vi "rsscope_core_global.vi"() -> ()   [LabVIEW 2018] (continued)
"Supported Models"="", "Instrument Options"="", "Flags"=0, "Help"="Adds additional time limitation to the pattern definition.\n\nAvailable Repeated Capabilities:\nNone\n\nRemote-control command(s):\nTRIGger<m>:PATTern:MODE"}, {"Level"=3, "Class Only"=FALSE, "Identifier"="RSSCOPE_ATTR_PATTERN_TIMEOUT_MODE", "Descriptive Name"="Pattern Timeout Mode", "Data Type"=0, "Command"="TRIG:PATT:TIM:MODE", "Access"=2, "Range Table"="rsscope_rngPatternTimeoutMode", "Read Callback"="", "Write Callback"="", "Supported Models"="", "Instrument Options"="", "Flags"=0, "Help"="Defines the condition for the timeout.\n\nAvailable Repeated Capabilities:\nNone\n\nRemote-control command(s):\nTRIGger<m>:PATTern:TIMeout:MODE"}, {"Level"=3, "Class Only"=FALSE, "Identifier"="RSSCOPE_ATTR_PATTERN_TIMEOUT", "Descriptive Name"="Pattern Timeout", "Data Type"=1, "Command"="TRIG:PATT:TIM", "Access"=2, "Range Table"="rsscope_rngWidth", "Read Callback"="", "Write Callback"="", "Supported Models"="", "Instrument Options"="", "Flags"=0, "Help"="Defines how long the result of the pattern condition must be true or false.\n\nAvailable Repeated Capabilities:\nNone\n\nRemote-control command(s):\nTRIGger<m>:PATTern:TIMeout[:TIME]"}, {"Level"=3, "Class Only"=FALSE, "Identifier"="RSSCOPE_ATTR_PATTERN_CONDITION", "Descriptive Name"="Pattern Condition", "Data Type"=0, "Command"="TRIG:PATT:WIDT:RANG", "Access"=2, "Range Table"="rsscope_rngWidthCondition", "Read Callback"="", "Write Callback"="", "Supported Models"="", "Instrument Options"="", "Flags"=0, "Help"="Defines how the range of a pulse width is defined for keeping up the true result of the pattern condition.\n\nAvailable Repeated Capabilities:\nNone\n\nRemote-control command(s):\nTRIGger<m>:PATTern:WIDTh:RANGe"}, {"Level"=3, "Class Only"=FALSE, "Identifier"="RSSCOPE_ATTR_PATTERN_WIDTH", "Descriptive Name"="Pattern Width", "Data Type"=1, "Command"="TRIG:PATT:WIDT", "Access"=2, "Range Table"="rsscope_rngWidth", "Read Callback"="", "Write Callback"="", "Supported Models"="", "Instrument Options"="", "Flags"=0, "Help"="For the ranges &apos;Within&apos; and &apos;Outside&apos;, the width defines the center of a range which is defined by the limits &apos;Delta&apos;.\nFor the ranges &apos;Shorter&apos; and &apos;Longer&apos;, the width defines the maximum and minimum pulse width, respectively.\n\nAvailable Repeated Capabilities:\nNone\n\nRemote-control command(s):\nTRIGger<m>:PATTern:WIDTh[:WIDTh]"}, {"Level"=3, "Class Only"=FALSE, "Identifier"="RSSCOPE_ATTR_PATTERN_DELTA", "Descriptive Name"="Pattern Delta", "Data Type"=1, "Command"="TRIG:PATT:WIDT:DELT", "Access"=2, "Range Table"="", "Read Callback"="", "Write Callback"="", "Supported Models"="", "Instrument Options"="", "Flags"=0, "Help"="Defines a time range around the width value.\n\nAvailable Repeated Capabilities:\nNone\n\nRemote-control command(s):\nTRIGger<m>:PATTern:WIDTh:DELTa"}, {"Level"=2, "Class Only"=TRUE, "Identifier"="", "Descriptive Name"="Serial Pattern Triggering", "Data Type"=0, "Command"="", "Access"=0, "Range Table"="", "Read Callback"="", "Write Callback"="", "Supported Models"="", "Instrument Options"="", "Flags"=0, "Help"="The serial pattern event is used to trigger on signals with serial data patterns in relation to a clock signal - for example, on bus signals like the I2C bus. For convenient and comprehensive triggering on specific serial data, options for serial protocol analysis are provided.\n\nThe serial pattern trigger is only available for the A-event (Suffix = 1)."}, {"Level"=3, "Class Only"=FALSE, "Identifier"="RSSCOPE_ATTR_SERIAL_PATTERN_SOURCE", "Descriptive Name"="Serial Pattern Source", "Data Type"=0, "Command"="TRIG:SPAT:CSO", "Access"=2, "Range Table"="RsScope_rngClockSource", "Read Callback"="", "Write Callback"="", "Supported Models"="", "Instrument Options"="", "Flags"=0, "Help"="Defines the input channel of the clock signal.\n\nAvailable Repeated Capabilities:\nNone\n\nRemote-control command(s):\nTRIGger<m>:SPATtern:CSOurce[:VALue]"}, {"Level"=3, "Class Only"=FALSE, "Identifier"="RSSCOPE_ATTR_SERIAL_PATTERN_LEVEL", "Descriptive Name"="Serial Pattern Level", "Data Type"=1, "Command"="TRIG:SPAT:CSO:LEV", "Access"=2, "Range Table"="", "Read Callback"="", "Write Callback"="", "Supported Models"="", "Instrument Options"="", "Flags"=0, "Help"="Defines the voltage level for the clock signal.\n\nAvailable Repeated Capabilities:\nNone\n\nRemote-control command(s):\nTRIGger<m>:SPATtern:CSOurce:LEVel"}, {"Level"=3, "Class Only"=FALSE, "Identifier"="RSSCOPE_ATTR_SERIAL_PATTERN", "Descriptive Name"="Serial Pattern", "Data Type"=2, "Command"="TRIG:SPAT:PATT", "Access"=2, "Range Table"="", "Read Callback"="", "Write Callback"="", "Supported Models"="", "Instrument Options"="", "Flags"=0, "Help"="The pattern contains the bits of the serial data to be found in the data stream. The maximum length of the pattern is 128 bit. You can enter the pattern in binary or hexadecimal format.\n\nAvailable Repeated Capabilities:\nNone\n\nRemote-control command(s):\nTRIGger<m>:SPATtern:PATTern"}, {"Level"=3, "Class Only"=FALSE, "Identifier"="RSSCOPE_ATTR_SERIAL_PATTERN_POLARITY", "Descriptive Name"="Serial Pattern Polarity", "Data Type"=0, "Command"="TRIG:SPAT:CSO:EDGE", "Access"=2, "Range Table"="rsscope_rngPolarity", "Read Callback"="", "Write Callback"="", "Supported Models"="", "Instrument Options"="", "Flags"=0, "Help"="Together with the clock level, the clock edge defines the point in time when the state of the data signal is checked.\n\nAvailable Repeated Capabilities:\nNone\n\nRemote-control command(s):\nTRIGger<m>:SPATtern:CSOurce:EDGE"}, {"Level"=3, "Class Only"=FALSE, "Identifier"="RSSCOPE_ATTR_SERIAL_PATTERN_TYPE", "Descriptive Name"="Serial Pattern Type", "Data Type"=0, "Command"="TRIG:SERP:PTMD", "Access"=2, "Range Table"="RsScope_rngSerialPatternType", "Read Callback"="", "Write Callback"="", "Supported Models"="RTP", "Instrument Options"="K140|K141", "Flags"=0, "Help"="Selects the pattern type for the serial pattern trigger.\n\nAvailable Repeated Capabilities:\nNone\n\nRemote-control command(s):\nTRIGger<m>:SERPattern:PTMDe"}, {"Level"=3, "Class Only"=TRUE, "Identifier"="", "Descriptive Name"="Single/Dual Bit", "Data Type"=0, "Command"="", "Access"=0, "Range Table"="", "Read Callback"="", "Write Callback"="", "Supported Models"="", "Instrument Options"="", "Flags"=0, "Help"="This class contains attributes for configuring single or dual bit trigger patterns on the R&S RTP-K140/-K141."}, {"Level"=4, "Class Only"=FALSE, "Identifier"="RSSCOPE_ATTR_SERIAL_PATTERN_BIT_PATTERN_A", "Descriptive Name"="Serial Pattern Bit Pattern A", "Data Type"=2, "Command"="TRIG:SERP:BITP:APAT", "Access"=2, "Range Table"="", "Read Callback"="", "Write Callback"="rsscope_FormatSearchNameString_WriteCallback.vi", "Supported Models"="RTP", "Instrument Options"="K140|K141", "Flags"=0, "Help"="Defines the bit pattern, or bit pattern A if RSSCOPE_ATTR_SERIAL_PATTERN_TYPE is set to SBP or DBP.\n\nAvailable Repeated Capabilities:\nNone\n\nRemote-control command(s):\nTRIGger<m>:SERPattern:BITPattern<n>:APATtern"}, {"Level"=4, "Class Only"=FALSE, "Identifier"="RSSCOPE_ATTR_SERIAL_PATTERN_BIT_PATTERN_B", "Descriptive Name"="Serial Pattern Bit Pattern B", "Data Type"=2, "Command"="TRIG:SERP:BITP:BPAT", "Access"=2, "Range Table"="", "Read Callback"="", "Write Callback"="rsscope_FormatSearchNameString_WriteCallback.vi", "Supported Models"="RTP", "Instrument Options"="K140|K141", "Flags"=0, "Help"="Defines the bit pattern B, if RSSCOPE_ATTR_SERIAL_PATTERN_TYPE is set to DBP.\n\nAvailable Repeated Capabilities:\nNone\n\nRemote-control command(s):\nTRIGger<m>:SERPattern:BITPattern<n>:BPATtern"}, {"Level"=4, "Class Only"=FALSE, "Identifier"="RSSCOPE_ATTR_SERIAL_PATTERN_BIT_PATTERN_LENGTH_A", "Descriptive Name"="Serial Pattern Bit Pattern Length A", "Data Type"=0, "Command"="TRIG:SERP:BITP:PTAL", "Access"=2, "Range Table"="RsScope_rngBitPatternLength", "Read Callback"="", "Write Callback"="", "Supported Models"="RTP", "Instrument Options"="K140|K141", "Flags"=0, "Help"="Sets the length of the bit pattern A.\n\nAvailable Repeated Capabilities:\nNone\n\nRemote-control command(s):\nTRIGger<m>:SERPattern:BITPattern<n>:PTALength"}, {"Level"=4, "Class Only"=FALSE, "Identifier"="RSSCOPE_ATTR_SERIAL_PATTERN_BIT_PATTERN_LENGTH_B", "Descriptive Name"="Serial Pattern Bit Pattern Length B", "Data Type"=0, "Command"="TRIG:SERP:BITP:PTBL", "Access"=2, "Range Table"="RsScope_rngBitPatternLength", "Read Callback"="", "Write Callback"="", "Supported Models"="RTP", "Instrument Options"="K140|K141", "Flags"=0, "Help"="Sets the length of the bit pattern B.\n\nAvailable Repeated Capabilities:\nNone\n\nRemote-control command(s):\nTRIGger<m>:SERPattern:BITPattern<n>:PTBLength"}, {"Level"=3, "Class Only"=TRUE, "Identifier"="", "Descriptive Name"="Complex Word", "Data Type"=0, "Command"="", "Access"=0, "Range Table"="", "Read Callback"="", "Write Callback"="", "Supported Models"="", "Instrument Options"="", "Flags"=0, "Help"="This class contains attributes for configuring complex word trigger patterns on the R&S RTP-K140/-K141."}, {"Level"=4, "Class Only"=FALSE, "Identifier"="RSSCOPE_ATTR_SERIAL_PATTERN_COMPLEX_WORD_ALIGNMENT_TYPE", "Descriptive Name"="Serial Pattern Complex Word Alignment Type", "Data Type"=0, "Command"="TRIG:SERP:COMP:SOFS", "Access"=2, "Range Table"="RsScope_rngComplexWordAlignmentType", "Read Callback"="", "Write Callback"="", "Supported Models"="RTP", "Instrument Options"="K140|K141", "Flags"=0, "Help"="Selects if the alignment for the complex word pattern triggering is done on a pattern value or on a defined timeout.\n\nAvailable Repeated Capabilities:\nNone\n\nRemote-control command(s):\nTRIGger<m>:SERPattern:COMPlex:SOFState"}, {"Level"=4, "Class Only"=FALSE, "Identifier"="RSSCOPE_ATTR_SERIAL_PATTERN_COMPLEX_WORD_ALIGNMENT_LENGTH", "Descriptive Name"="Serial Pattern Complex Word Alignment Length", "Data Type"=0, "Command"="TRIG:SERP:COMP:SOFL", "Access"=2, "Range Table"="RsScope_rngComplexWordLength", "Read Callback"="", "Write Callback"="", "Supported Models"="RTP", "Instrument Options"="K140|K141", "Flags"=0, "Help"="Sets the length of the pattern for the trigger alignment condition.\n\nAvailable Repeated Capabilities:\nNone\n\nRemote-control command(s):\nTRIGger<m>:SERPattern:COMPlex:SOFLength"}, {"Level"=4, "Class Only"=FALSE, "Identifier"="RSSCOPE_ATTR_SERIAL_PATTERN_COMPLEX_WORD_ALIGNMENT_PATTERN", "Descriptive Name"="Serial Pattern Complex Word Alignment Pattern", "Data Type"=2, "Command"="TRIG:SERP:COMP:SOFP", "Access"=2, "Range Table"="", "Read Callback"="", "Write Callback"="rsscope_FormatSearchNameString_WriteCallback.vi", "Supported Models"="RTP", "Instrument Options"="K140|K141", "Flags"=0, "Help"="Sets the bit pattern value for the trigger alignment condition, if RSSCOPE_ATTR_SERIAL_PATTERN_COMPLEX_WORD_ALIGNMENT_TYPE is set to PATTern.\n\nAvailable Repeated Capabilities:\nNone\n\nRemote-control command(s):\nTRIGger<m>:SERPattern:COMPlex:SOFPattern"}, {"Level"=4, "Class Only"=FALSE, "Identifier"="RSSCOPE_ATTR_SERIAL_PATTERN_COMPLEX_WORD_ALIGNMENT_TIMEOUT", "Descriptive Name"="Serial Pattern Complex Word Alignment Timeout", "Data Type"=1, "Command"="TRIG:SERP:COMP:SOFT", "Access"=2, "Range Table"="RsScope_rngComplexWordAlignmentTimeout", "Read Callback"="", "Write Callback"="", "Supported Models"="RTP", "Instrument Options"="K140|K141", "Flags"=0, "Help"="Sets the timeout, a duration that defines an idle mark, if RSSCOPE_ATTR_SERIAL_PATTERN_COMPLEX_WORD_ALIGNMENT_TYPE is set to TIMEout.\n\nAvailable Repeated Capabilities:\nNone\n\nRemote-control command(s):\nTRIGger<m>:SERPattern:COMPlex:SOFTimeout"}, {"Level"=4, "Class Only"=FALSE, "Identifier"="RSSCOPE_ATTR_SERIAL_PATTERN_COMPLEX_WORD_IDLE_RANGE", "Descriptive Name"="Serial Pattern Complex Word Idle Range", "Data Type"=0, "Command"="TRIG:SERP:COMP:IDLR", "Access"=2, "Range Table"="RsScope_rngComplexWordIdleRange", "Read Callback"="", "Write Callback"="", "Supported Models"="RTP", "Instrument Options"="K140|K141", "Flags"=0, "Help"="Selects if the timeout should be within the range or out of range.\n\nAvailable Repeated Capabilities:\nNone\n\nRemote-control command(s):\nTRIGger<m>:SERPattern:COMPlex:IDLRange"}, {"Level"=4, "Class Only"=FALSE, "Identifier"="RSSCOPE_ATTR_SERIAL_PATTERN_COMPLEX_WORD_LOGIC", "Descriptive Name"="Serial Pattern Complex Word Logic", "Data Type"=0, "Command"="TRIG:SERP:COMP:CLOG", "Access"=2, "Range Table"="RsScope_rngConditionAndOr", "Read Callback"="", "Write Callback"="", "Supported Models"="RTP", "Instrument Options"="K140|K141", "Flags"=0, "Help"="Selects the logic for the condition, if more than one pattern conditions are defined.\n\nAvailable Repeated Capabilities:\nNone\n\nRemote-control command(s):\nTRIGger<m>:SERPattern:COMPlex:CLOGic"}, {"Level"=4, "Class Only"=FALSE, "Identifier"="RSSCOPE_ATTR_SERIAL_PATTERN_COMPLEX_WORD_BIT_ORDER", "Descriptive Name"="Serial Pattern Complex Word Bit Order", "Data Type"=0, "Command"="TRIG:SERP:COMP:BORD", "Access"=2, "Range Table"="RsScope_rngComplexWordBitOrder", "Read Callback"="", "Write Callback"="", "Supported Models"="RTP", "Instrument Options"="K140|K141", "Flags"=0, "Help"="Sets the most significant bit (MSB) or least significant bit (LSB) to define the data bit order.\n\nAvailable Repeated Capabilities:\nNone\n\nRemote-control command(s):\nTRIGger<m>:SERPattern:COMPlex:BORDer"}, {"Level"=4, "Class Only"=FALSE, "Identifier"="RSSCOPE_ATTR_SERIAL_PATTERN_COMPLEX_WORD_CONDITION_ENABLED", "Descriptive Name"="Serial Pattern Complex Word Condition Enabled", "Data Type"=3, "Command"="TRIG:SERP:COMP:PATT{ComplexCondition}:ENAB", "Access"=2, "Range Table"="", "Read Callback"="", "Write Callback"="", "Supported Models"="RTP", "Instrument Options"="K140|K141", "Flags"=0, "Help"="Enables a new pattern condition.\n\nAvailable Repeated Capabilities:\nComplexCondition: Complex1, Complex2, Complex3, Complex4\r\n\nRemote-control command(s):\nTRIGger<m>:SERPattern:COMPlex:PATTern<n>:ENABle"}, {"Level"=4, "Class Only"=FALSE, "Identifier"="RSSCOPE_ATTR_SERIAL_PATTERN_COMPLEX_WORD_BIT_OFFSET", "Descriptive Name"="Serial Pattern Complex Word Bit Offset", "Data Type"=0, "Command"="TRIG:SERP:COMP:PATT{ComplexCondition}:BOFF", "Access"=2, "Range Table"="RsScope_rngComplexWordBitOffset", "Read Callback"="", "Write Callback"="", "Supported Models"="RTP", "Instrument Options"="K140|K141", "Flags"=0, "Help"="Sets the number of arbitrary bits between the first bit after the frame id and the first bit of the word pattern.\n\nAvailable Repeated Capabilities:\nComplexCondition: Complex1, Complex2, Complex3, Complex4\r\n\nRemote-control command(s):\nTRIGger<m>:SERPattern:COMPlex:PATTern<n>:BOFFset"}, {"Level"=4, "Class Only"=FALSE, "Identifier"="RSSCOPE_ATTR_SERIAL_PATTERN_COMPLEX_WORD_PATTERN_LENGTH", "Descriptive Name"="Serial Pattern Complex Word Pattern Length", "Data Type"=0, "Command"="TRIG:SERP:COMP:PATT{ComplexCondition}:PATL", "Access"=2, "Range Table"="RsScope_rngComplexWordPatternLength", "Read Callback"="", "Write Callback"="", "Supported Models"="RTP", "Instrument Options"="K140|K141", "Flags"=0, "Help"="Sets the word pattern length in bits. The maximal bit length of all selected pattern conditions is 160 bits.\n\nAvailable Repeated Capabilities:\nComplexCondition: Complex1, Complex2, Complex3, Complex4\r\n\nRemote-control command(s):\nTRIGger<m>:SERPattern:COMPlex:PATTern<n>:PATLength"}, {"Level"=4, "Class Only"=FALSE, "Identifier"="RSSCOPE_ATTR_SERIAL_PATTERN_COMPLEX_WORD_SEARCH_RANGE", "Descriptive Name"="Serial Pattern Complex Word Search Range", "Data Type"=0, "Command"="TRIG:SERP:COMP:PATT{ComplexCondition}:SRNG", "Access"=2, "Range Table"="RsScope_rngComplexWordSearchRange", "Read Callback"="", "Write Callback"="", "Supported Models"="RTP", "Instrument Options"="K140|K141", "Flags"=0, "Help"="Sets the search range of the word pattern.\n\nAvailable Repeated Capabilities:\nComplexCondition: Complex1, Complex2, Complex3, Complex4\r\n\nRemote-control command(s):\nTRIGger<m>:SERPattern:COMPlex:PATTern<n>:SRNGe"}, {"Level"=4, "Class Only"=FALSE, "Identifier"="RSSCOPE_ATTR_SERIAL_PATTERN_COMPLEX_WORD_PATTERN_CONDITION", "Descriptive Name"="Serial Pattern Complex Word Pattern Condition", "Data Type"=0, "Command"="TRIG:SERP:COMP:PATT{ComplexCondition}:PCON", "Access"=2, "Range Table"="RsScope_rngComplexWordPatternCondition", "Read Callback"="", "Write Callback"="", "Supported Models"="RTP", "Instrument Options"="K140|K141", "Flags"=0, "Help"="Sets the operator to define the exact position or range where the instrument looks for the specified pattern.\n\nAvailable Repeated Capabilities:\nComplexCondition: Complex1, Complex2, Complex3, Complex4\r\n\nRemote-control command(s):\nTRIGger<m>:SERPattern:COMPlex:PATTern<n>:PCONdition"}, {"Level"=4, "Class Only"=FALSE, "Identifier"="RSSCOPE_ATTR_SERIAL_PATTERN_COMPLEX_WORD_PATTERN", "Descriptive Name"="Serial Pattern Complex Word Pattern", "Data Type"=2, "Command"="TRIG:SERP:COMP:PATT{ComplexCondition}:FRPT", "Access"=2, "Range Table"="", "Read Callback"="", "Write Callback"="rsscope_FormatSearchNameString_WriteCallback.vi", "Supported Models"="RTP", "Instrument Options"="K140|K141", "Flags"=0, "Help"="Sets the pattern or a start value of a pattern range.\n\nAvailable Repeated Capabilities:\nComplexCondition: Complex1, Complex2, Complex3, Complex4\r\n\nRemote-control command(s):\nTRIGger<m>:SERPattern:COMPlex:PATTern<n>:FRPTtern"}, {"Level"=4, "Class Only"=FALSE, "Identifier"="RSSCOPE_ATTR_SERIAL_PATTERN_COMPLEX_WORD_PATTERN_RANGE_END", "Descriptive Name"="Serial Pattern Complex Word Pattern Range End", "Data Type"=2, "Command"="TRIG:SERP:COMP:PATT{ComplexCondition}:TOPT", "Access"=2, "Range Table"="", "Read Callback"="", "Write Callback"="", "Supported Models"="RTP", "Instrument Options"="K140|K141", "Flags"=0, "Help"="Sets the end value of a pattern range if RSSCOPE_ATTR_SERIAL_PATTERN_COMPLEX_WORD_PATTERN_CONDITION is set to In Range or Out Of Range.\n\nAvailable Repeated Capabilities:\nComplexCondition: Complex1, Complex2, Complex3, Complex4\r\n\nRemote-control command(s):\nTRIGger<m>:SERPattern:COMPlex:PATTern<n>:TOPTtern"}, {"Level"=3, "Class Only"=TRUE, "Identifier"="", "Descriptive Name"="PRBS", "Data Type"=0, "Command"="", "Access"=0, "Range Table"="", "Read Callback"="", "Write Callback"="", "Supported Models"="", "Instrument Options"="", "Flags"=0, "Help"="This class contains attributes for configuring PRBS sequences on the R&S RTP-K140/-K141."}, {"Level"=4, "Class Only"=FALSE, "Identifier"="RSSCOPE_ATTR_SERIAL_PATTERN_PRBS_ERROR_RATE", "Descriptive Name"="Serial Pattern PRBS Error Rate", "Data Type"=1, "Command"="TRIG:SERP:PRBS:ERAT", "Access"=2, "Range Table"="RsScope_rngPRBSErrorRate", "Read Callback"="", "Write Callback"="", "Supported Models"="RTP", "Instrument Options"="K140|K141", "Flags"=0, "Help"="Sets the bit error rate for the PRBS sequence.\n\nAvailable Repeated Capabilities:\nNone\n\nRemote-control command(s):\nTRIGger<m>:SERPattern:PRBS:ERATe"}, {"Level"=4, "Class Only"=FALSE, "Identifier"="RSSCOPE_ATTR_SERIAL_PATTERN_PRBS_NOMINAL_BIT_RATE", "Descriptive Name"="Serial Pattern PRBS Nominal Bit Rate", "Data Type"=1, "Command"="TRIG:SERP:PRBS:NBRT", "Access"=2, "Range Table"="RsScope_rngPRBSNominalBitRate", "Read Callback"="", "Write Callback"="", "Supported Models"="RTP", "Instrument Options"="K140|K141", "Flags"=0, "Help"="Sets the nominal bit error rate for the PRBS sequence. It corresponds to the data rate of the data stream from which the clock is to be recovered.\n\nAvailable Repeated Capabilities:\nNone\n\nRemote-control command(s):\nTRIGger<m>:SERPattern:PRBS:NBRTe"}, {"Level"=4, "Class Only"=FALSE, "Identifier"="RSSCOPE_ATTR_SERIAL_PATTERN_PRBS_SEQUENCE", "Descriptive Name"="Serial Pattern PRBS Sequence", "Data Type"=0, "Command"="TRIG:SERP:PRBS:PSEQ", "Access"=2, "Range Table"="RsScope_rngPRBSSequence", "Read Callback"="", "Write Callback"="", "Supported Models"="RTP", "Instrument Options"="K140|K141", "Flags"=0, "Help"="Selects a predefined pseudorandom binary sequence.\n\nAvailable Repeated Capabilities:\nNone\n\nRemote-control command(s):\nTRIGger<m>:SERPattern:PRBS:PSEQuence"}, {"Level"=3, "Class Only"=TRUE, "Identifier"="", "Descriptive Name"="8b/10b", "Data Type"=0, "Command"="", "Access"=0, "Range Table"="", "Read Callback"="", "Write Callback"="", "Supported Models"="", "Instrument Options"="", "Flags"=0, "Help"="This class contains attributes for configuring an 8b/10b pattern on the R&S RTP-K140/-K141."}, {"Level"=4, "Class Only"=FALSE, "Identifier"="RSSCOPE_ATTR_SERIAL_PATTERN_EBTB_ALIGNMENT_SYMBOL", "Descriptive Name"="Serial Pattern EbTb Alignment Symbol", "Data Type"=0, "Command"="TRIG:SERP:EBTB:ALIG", "Access"=2, "Range Table"="RsScope_rngEbTbAlignmentSymbol", "Read Callback"="", "Write Callback"="", "Supported Models"="RTP", "Instrument Options"="K140|K141", "Flags"=0, "Help"="Selects one of the comma control symbols used for synchronization. The alignment symbol cannot be reused in a pattern.\n\nAvailable Repeated Capabilities:\nNone\n\nRemote-control command(s):\nTRIGger<m>:SERPattern:EBTB:ALIGnment"}, {"Level"=4, "Class Only"=FALSE, "Identifier"="RSSCOPE_ATTR_SERIAL_PATTERN_EBTB_SCRAMBLING", "Descriptive Name"="Serial Pattern EbTb Scrambling", "Data Type"=0, "Command"="TRIG:SERP:EBTB:SCRM", "Access"=2, "Range Table"="RsScope_rngEbTbScrambling", "Read Callback"="", "Write Callback"="", "Supported Models"="RTP", "Instrument Options"="K140|K141", "Flags"=0, "Help"="Selects if the data is scrambled or unscrambled.\n\nAvailable Repeated Capabilities:\nNone\n\nRemote-control command(s):\nTRIGger<m>:SERPattern:EBTB:SCRMble"}, {"Level"=4, "Class Only"=FALSE, "Identifier"="RSSCOPE_ATTR_SERIAL_PATTERN_EBTB_KD_SYMBOL", "Descriptive Name"="Serial Pattern EbTb K/D Symbol", "Data Type"=2, "Command"="TRIG:SERP:EBTB:SYMB{EbTbSymbol}:KDSY", "Access"=2, "Range Table"="", "Read Callback"="", "Write Callback"="", "Supported Models"="RTP", "Instrument Options"="K140|K141", "Flags"=0, "Help"="Sets the data character (Dx.y) or the control character (Kx.y). This cannot be the same as the alignment symbol RSSCOPE_ATTR_SERIAL_PATTERN_EBTB_ALIGNMENT_SYMBOL.\n\nAvailable Repeated Capabilities:\nEbTbSymbol: EbTb1, EbTb2, EbTb3, EbTb4, EbTb5, EbTb6, EbTb7, EbTb8, EbTb9, EbTb10, EbTb11, EbTb12, EbTb13, EbTb14, EbTb15, EbTb16\r\n\nRemote-control command(s):\nTRIGger<m>:SERPattern:EBTB:SYMBols<n>:KDSYmbol"}, {"Level"=4, "Class Only"=FALSE, "Identifier"="RSSCOPE_ATTR_SERIAL_PATTERN_EBTB_EIGHT_BIT_VALUE", "Descriptive Name"="Serial Pattern EbTb Eight Bit Value", "Data Type"=2, "Command"="TRIG:SERP:EBTB:SYMB{EbTbSymbol}:EBIT", "Access"=2, "Range Table"="", "Read Callback"="", "Write Callback"="", "Supported Models"="RTP", "Instrument Options"="K140|K141", "Flags"=0, "Help"="Sets the 8b bit value.\n\nAvailable Repeated Capabilities:\nEbTbSymbol: EbTb1, EbTb2, EbTb3, EbTb4, EbTb5, EbTb6, EbTb7, EbTb8, EbTb9, EbTb10, EbTb11, EbTb12, EbTb13, EbTb14, EbTb15, EbTb16\r\n\nRemote-control command(s):\nTRIGger<m>:SERPattern:EBTB:SYMBols<n>:EBIT"}, {"Level"=4, "Class Only"=FALSE, "Identifier"="RSSCOPE_ATTR_SERIAL_PATTERN_EBTB_TEN_BIT_D_PLUS", "Descriptive Name"="Serial Pattern EbTb Ten Bit D Plus", "Data Type"=2, "Command"="TRIG:SERP:EBTB:SYMB{EbTbSymbol}:DPL?", "Access"=0, "Range Table"="", "Read Callback"="", "Write Callback"="", "Supported Models"="RTP", "Instrument Options"="K140|K141", "Flags"=0, "Help"="Returns the value for the positive running disparity RD+.\n\nAvailable Repeated Capabilities:\nEbTbSymbol: EbTb1, EbTb2, EbTb3, EbTb4, EbTb5, EbTb6, EbTb7, EbTb8, EbTb9, EbTb10, EbTb11, EbTb12, EbTb13, EbTb14, EbTb15, EbTb16\r\n\nRemote-control command(s):\nTRIGger<m>:SERPattern:EBTB:SYMBols<n>:DPLus?"}, {"Level"=4, "Class Only"=FALSE, "Identifier"="RSSCOPE_ATTR_SERIAL_PATTERN_EBTB_TEN_BIT_D_MINUS", "Descriptive Name"="Serial Pattern EbTb Ten Bit D Minus", "Data Type"=2, "Command"="TRIG:SERP:EBTB:SYMB{EbTbSymbol}:DMIN?", "Access"=0, "Range Table"="", "Read Callback"="", "Write Callback"="", "Supported Models"="RTP", "Instrument Options"="K140|K141", "Flags"=0, "Help"="Returns the value for the negative running disparity RD-.\n\nAvailable Repeated Capabilities:\nEbTbSymbol: EbTb1, EbTb2, EbTb3, EbTb4, EbTb5, EbTb6, EbTb7, EbTb8, EbTb9, EbTb10, EbTb11, EbTb12, EbTb13, EbTb14, EbTb15, EbTb16\r\n\nRemote-control command(s):\nTRIGger<m>:SERPattern:EBTB:SYMBols<n>:DMINus?"}, {"Level"=4, "Class Only"=FALSE, "Identifier"="RSSCOPE_ATTR_SERIAL_PATTERN_EBTB_APPEND_ROW", "Descriptive Name"="Serial Pattern EbTb Append Row", "Data Type"=4, "Command"="TRIG:SERP:EBTB:APP", "Access"=1, "Range Table"="", "Read Callback"="", "Write Callback"="", "Supported Models"="RTP", "Instrument Options"="K140|K141", "Flags"=0, "Help"="Creates an empty row and adds it to the end of the active symbol description in the 8b/10b table.\n\nAvailable Repeated Capabilities:\nNone\n\nRemote-control command(s):\nTRIGger<m>:SERPattern:EBTB:APPend"}, {"Level"=4, "Class Only"=FALSE, "Identifier"="RSSCOPE_ATTR_SERIAL_PATTERN_EBTB_ROW_COUNT", "Descriptive Name"="Serial Pattern EbTb Row Count", "Data Type"=0, "Command"="TRIG:SERP:EBTB:COUN?", "Access"=0, "Range Table"="", "Read Callback"="", "Write Callback"="", "Supported Models"="RTP", "Instrument Options"="K140|K141", "Flags"=0, "Help"="Queries the number of 8b/10b symbols.\n\nAvailable Repeated Capabilities:\nNone\n\nRemote-control command(s):\nTRIGger<m>:SERPattern:EBTB:COUNt?"}, {"Level"=4, "Class Only"=FALSE, "Identifier"="RSSCOPE_ATTR_SERIAL_PATTERN_EBTB_CLEAR_TABLE", "Descriptive Name"="Serial Pattern EbTb Clear Table", "Data Type"=4, "Command"="TRIG:SERP:EBTB:CLE", "Access"=1, "Range Table"="", "Read Callback"="", "Write Callback"="", "Supported Models"="RTP", "Instrument Options"="K140|K141", "Flags"=0, "Help"="Removes all entries from the 8b/10b table.\n\nAvailable Repeated Capabilities:\nNone\n\nRemote-control command(s):\nTRIGger<m>:SERPattern:EBTB:CLEar"}, {"Level"=4, "Class Only"=FALSE, "Identifier"="RSSCOPE_ATTR_SERIAL_PATTERN_EBTB_DISPARITY_ERROR_ENABLED", "Descriptive Name"="Serial Pattern EbTb Disparity Error Enabled", "Data Type"=3, "Command"="TRIG:SERP:EBTB:ERR:DISP", "Access"=2, "Range Table"="", "Read Callback"="", "Write Callback"="", "Supported Models"="RTP", "Instrument Options"="K140|K141", "Flags"=0, "Help"="Enables triggering on disparity errors.\n\nAvailable Repeated Capabilities:\nNone\n\nRemote-control command(s):\nTRIGger<m>:SERPattern:EBTB:ERRor<n>:DISParity"}, {"Level"=4, "Class Only"=FALSE, "Identifier"="RSSCOPE_ATTR_SERIAL_PATTERN_EBTB_SYMBOL_ERROR_ENABLED", "Descriptive Name"="Serial Pattern EbTb Symbol Error Enabled", "Data Type"=3, "Command"="TRIG:SERP:EBTB:ERR:SYMB", "Access"=2, "Range Table"="", "Read Callback"="", "Write Callback"="", "Supported Models"="RTP", "Instrument Options"="K140|K141", "Flags"=0, "Help"="Enables triggering on symbol errors.\n\nAvailable Repeated Capabilities:\nNone\n\nRemote-control command(s):\nTRIGger<m>:SERPattern:EBTB:ERRor<n>:SYMBol"}, {"Level"=4, "Class Only"=FALSE, "Identifier"="RSSCOPE_ATTR_SERIAL_PATTERN_EBTB_FRAME_ID", "Descriptive Name"="Serial Pattern EbTb Frame ID", "Data Type"=0, "Command"="TRIG:SERP:EBTB:FID", "Access"=2, "Range Table"="RsScope_rngFrameID", "Read Callback"="", "Write Callback"="", "Supported Models"="RTP", "Instrument Options"="K140|K141", "Flags"=0, "Help"="Selects the frame ID.\n\nAvailable Repeated Capabilities:\nNone\n\nRemote-control command(s):\nTRIGger<m>:SERPattern:EBTB:FID"}, {"Level"=3, "Class Only"=TRUE, "Identifier"="", "Descriptive Name"="127b/132b", "Data Type"=0, "Command"="", "Access"=0, "Range Table"="", "Read Callback"="", "Write Callback"="", "Supported Models"="", "Instrument Options"="", "Flags"=0, "Help"="This class contains attributes for configuring a 127b/132b pattern on the R&S RTP-K140/-K141."}, {"Level"=4, "Class Only"=FALSE, "Identifier"="RSSCOPE_ATTR_SERIAL_PATTERN_I32B_ALIGNMENT_PATTERN", "Descriptive Name"="Serial Pattern I32B Alignment Pattern", "Data Type"=2, "Command"="TRIG:SERP:I32B:APAT", "Access"=2, "Range Table"="", "Read Callback"="", "Write Callback"="", "Supported Models"="RTP", "Instrument Options"="K140|K141", "Flags"=0, "Help"="Sets the alignment pattern.\n\nAvailable Repeated Capabilities:\nNone\n\nRemote-control command(s):\nTRIGger<m>:SERPattern:I32B:APATtern"}, {"Level"=4, "Class Only"=FALSE, "Identifier"="RSSCOPE_ATTR_SERIAL_PATTERN_I32B_SKIP_START", "Descriptive Name"="Serial Pattern I32B Skip Start", "Data Type"=2, "Command"="TRIG:SERP:I32B:SSTR", "Access"=2, "Range Table"="", "Read Callback"="", "Write Callback"="", "Supported Models"="RTP", "Instrument Options"="K140|K141", "Flags"=0, "Help"="Sets the start skip value.\n\nAvailable Repeated Capabilities:\nNone\n\nRemote-control command(s):\nTRIGger<m>:SERPattern:I32B:SSTR"}, {"Level"=4, "Class Only"=FALSE, "Identifier"="RSSCOPE_ATTR_SERIAL_PATTERN_I32B_SKIP_END", "Descriptive Name"="Serial Pattern I32B Skip End", "Data Type"=2, "Command"="TRIG:SERP:I32B:SSTP", "Access"=2, "Range Table"="", "Read Callback"="", "Write Callback"="", "Supported Models"="RTP", "Instrument Options"="K140|K141", "Flags"=0, "Help"="Sets the skip end symbol.\n\nAvailable Repeated Capabilities:\nNone\n\nRemote-control command(s):\nTRIGger<m>:SERPattern:I32B:SSTP"}, {"Level"=4, "Class Only"=FALSE, "Identifier"="RSSCOPE_ATTR_SERIAL_PATTERN_I32B_SKIP_BYTES", "Descriptive Name"="Serial Pattern I32B Skip Bytes", "Data Type"=0, "Command"="TRIG:SERP:I32B:SKAF", "Access"=2, "Range Table"="RsScope_rngI32BSkipBytes", "Read Callback"="", "Write Callback"="", "Supported Models"="RTP", "Instrument Options"="K140|K141", "Flags"=0, "Help"="Sets the skip bytes symbols send after a skip end symbol.\n\nAvailable Repeated Capabilities:\nNone\n\nRemote-control command(s):\nTRIGger<m>:SERPattern:I32B:SKAFter"}, {"Level"=4, "Class Only"=FALSE, "Identifier"="RSSCOPE_ATTR_SERIAL_PATTERN_I32B_TYPE", "Descriptive Name"="Serial Pattern I32B Type", "Data Type"=0, "Command"="TRIG:SERP:I32B:SYMT", "Access"=2, "Range Table"="RsScope_rngI32BType", "Read Callback"="", "Write Callback"="", "Supported Models"="RTP", "Instrument Options"="K140|K141", "Flags"=0, "Help"="Selects the type of pattern, control block or the data block.\n\nAvailable Repeated Capabilities:\nNone\n\nRemote-control command(s):\nTRIGger<m>:SERPattern:I32B:SYMType"}, {"Level"=4, "Class Only"=FALSE, "Identifier"="RSSCOPE_ATTR_SERIAL_PATTERN_I32B_PATTERN", "Descriptive Name"="Serial Pattern I32B Pattern", "Data Type"=2, "Command"="TRIG:SERP:I32B:PATT", "Access"=2, "Range Table"="", "Read Callback"="", "Write Callback"="", "Supported Models"="RTP", "Instrument Options"="K140|K141", "Flags"=0, "Help"="Defines the control block or data block pattern in binary or hex format.\n\nAvailable Repeated Capabilities:\nNone\n\nRemote-control command(s):\nTRIGger<m>:SERPattern:I32B:PATTern"}, {"Level"=3, "Class Only"=TRUE, "Identifier"="", "Descriptive Name"="128b/132b", "Data Type"=0, "Command"="", "Access"=0, "Range Table"="", "Read Callback"="", "Write Callback"="", "Supported Models"="", "Instrument Options"="", "Flags"=0, "Help"="This class contains attributes for configuring a 128b/132b pattern on the R&S RTP-K140/-K141."}, {"Level"=4, "Class Only"=FALSE, "Identifier"="RSSCOPE_ATTR_SERIAL_PATTERN_I30B_ALIGNMENT_PATTERN", "Descriptive Name"="Serial Pattern I30B Alignment Pattern", "Data Type"=6, "Command"="TRIG{Trigger}:SERP:I30B:APAT", "Access"=2, "Range Table"="", "Read Callback"="", "Write Callback"="", "Supported Models"="RTP", "Instrument Options"="K140|K141", "Flags"=0, "Help"="Sets the alignment pattern.\n\nAvailable Repeated Capabilities:\nTrigger: TrigA, TrigB, TrigR\r\n\nRemote-control command(s):\nTRIGger<m>:SERPattern:I30B:APATtern"}, {"Level"=4, "Class Only"=FALSE, "Identifier"="RSSCOPE_ATTR_SERIAL_PATTERN_I30B_SKIP_START", "Descriptive Name"="Serial Pattern I30B Skip Start", "Data Type"=6, "Command"="TRIG{Trigger}:SERP:I30B:SSTR", "Access"=2, "Range Table"="", "Read Callback"="", "Write Callback"="", "Supported Models"="RTP", "Instrument Options"="K140|K141", "Flags"=0, "Help"="Sets the start skip value.\n\nAvailable Repeated Capabilities:\nTrigger: TrigA, TrigB, TrigR\r\n\nRemote-control command(s):\nTRIGger<m>:SERPattern:I30B:SSTR"}, {"Level"=4, "Class Only"=FALSE, "Identifier"="RSSCOPE_ATTR_SERIAL_PATTERN_I30B_SKIP_END", "Descriptive Name"="Serial Pattern I30B Skip End", "Data Type"=6, "Command"="TRIG{Trigger}:SERP:I30B:SSTP", "Access"=2, "Range Table"="", "Read Callback"="", "Write Callback"="", "Supported Models"="RTP", "Instrument Options"="K140|K141", "Flags"=0, "Help"="Sets the skip end symbol.\n\nAvailable Repeated Capabilities:\nTrigger: TrigA, TrigB, TrigR\r\n\nRemote-control command(s):\nTRIGger<m>:SERPattern:I30B:SSTP"}, {"Level"=4, "Class Only"=FALSE, "Identifier"="RSSCOPE_ATTR_SERIAL_PATTERN_I30B_SKIP_BYTES", "Descriptive Name"="Serial Pattern I30B Skip Bytes", "Data Type"=0, "Command"="TRIG{Trigger}:SERP:I30B:SKAF", "Access"=2, "Range Table"="RsScope_rngI30BSkipBytes", "Read Callback"="", "Write Callback"="", "Supported Models"="RTP", "Instrument Options"="K140|K141", "Flags"=0, "Help"="Sets the skip bytes symbols send after a skip end symbol.\n\nAvailable Repeated Capabilities:\nTrigger: TrigA, TrigB, TrigR\r\n\nRemote-control command(s):\nTRIGger<m>:SERPattern:I30B:SKAFter"}, {"Level"=4, "Class Only"=FALSE, "Identifier"="RSSCOPE_ATTR_SERIAL_PATTERN_I30B_TYPE", "Descriptive Name"="Serial Pattern I30B Type", "Data Type"=0, "Command"="TRIG{Trigger}:SERP:I30B:SYMT", "Access"=2, "Range Table"="RsScope_rngI30BType", "Read Callback"="", "Write Callback"="", "Supported Models"="RTP", "Instrument Options"="K140|K141", "Flags"=0, "Help"="Selects the type of pattern, control block or the data block.\n\nAvailable Repeated Capabilities:\nTrigger: TrigA, TrigB, TrigR\r\n\nRemote-control command(s):\nTRIGger<m>:SERPattern:I30B:SYMType"}, {"Level"=4, "Class Only"=FALSE, "Identifier"="RSSCOPE_ATTR_SERIAL_PATTERN_I30B_PATTERN", "Descriptive Name"="Serial Pattern I30B Pattern", "Data Type"=2, "Command"="TRIG{Trigger}:SERP:I30B:PATT", "Access"=2, "Range Table"="", "Read Callback"="", "Write Callback"="", "Supported Models"="RTP", "Instrument Options"="K140|K141", "Flags"=0, "Help"="Defines the OS or data block pattern in binary or hex format.\n\nAvailable Repeated Capabilities:\nTrigger: TrigA, TrigB, TrigR\r\n\nRemote-control command(s):\nTRIGger<m>:SERPattern:I30B:PATTern"}, {"Level"=2, "Class Only"=TRUE, "Identifier"="", "Descriptive Name"="NFC Trigger", "Data Type"=0, "Command"="", "Access"=0, "Range Table"="", "Read Callback"="", "Write Callback"="", "Supported Models"="", "Instrument Options"="", "Flags"=0, "Help"="Attributes that configures NFC Trigger"}, {"Level"=3, "Class Only"=FALSE, "Identifier"="RSSCOPE_ATTR_NFC_TRIGGER_TECHNOLOGY", "Descriptive Name"="NFC Trigger Technology", "Data Type"=0, "Command"="TRIGger1:NFC:TECH", "Access"=2, "Range Table"="rsscope_rngNFCTechnology", "Read Callback"="", "Write Callback"="", "Supported Models"="", "Instrument Options"="", "Flags"=0, "Help"="Selects the NFC technology, the communication protocol used by the input signal.\n\nAvailable Repeated Capabilities:\nNone\n\nRemote-control command(s):\nTRIGger<m>:NFC:TECHnology"}, {"Level"=3, "Class Only"=FALSE, "Identifier"="RSSCOPE_ATTR_NFC_TRIGGER_BIT_RATE", "Descriptive Name"="NFC Trigger Bit Rate", "Data Type"=0, "Command"="TRIGger1:NFC:BITR", "Access"=2, "Range Table"="rsscope_rngNFCTriggerBitRate", "Read Callback"="", "Write Callback"="", "Supported Models"="", "Instrument Options"="", "Flags"=0, "Help"="Sets the bit rate of the signal. \n\nFor NFC-A and NFC-B, the bit rate is always 106 kBit per second. For NFC-F, the bit rate can be either 212 or 424 kBit per second.\n\nAvailable Repeated Capabilities:\nNone\n\nRemote-control command(s):\nTRIGger<m>:NFC:BITRate"}, {"Level"=3, "Class Only"=FALSE, "Identifier"="RSSCOPE_ATTR_NFC_TRIGGER_EVENT", "Descriptive Name"="NFC Trigger Event", "Data Type"=0, "Command"="TRIGger1:NFC:EVEN", "Access"=2, "Range Table"="rsscope_rngNFCTriggerEvent", "Read Callback"="", "Write Callback"="", "Supported Models"="", "Instrument Options"="", "Flags"=0, "Help"="Sets the event to be triggered on.\n\nAvailable Repeated Capabilities:\nNone\n\nRemote-control command(s):\nTRIGger<m>:NFC:EVENt"}, {"Level"=2, "Class Only"=TRUE, "Identifier"="", "Descriptive Name"="TV Trigger", "Data Type"=0, "Command"="", "Access"=0, "Range Table"="", "Read Callback"="", "Write Callback"="", "Supported Models"="", "Instrument Options"="", "Flags"=0, "Help"="Attributes that configure the oscilloscope to trigger on TV signals."}, {"Level"=3, "Class Only"=FALSE, "Identifier"="RSSCOPE_ATTR_TV_TRIGGER_STANDARD", "Descriptive Name"="TV Trigger Standard", "Data Type"=0, "Command"="TRIG:TV:STAN", "Access"=2, "Range Table"="rsscope_rngConfigureTVTriggerStandard", "Read Callback"="", "Write Callback"="", "Supported Models"="", "Instrument Options"="", "Flags"=0, "Help"="Sets the TV standard.\n\nAvailable Repeated Capabilities:\nNone\n\nRemote-control command(s):\nTRIGger<m>:TV:STANdard"}, {"Level"=3, "Class Only"=FALSE, "Identifier"="RSSCOPE_ATTR_TV_TRIGGER_MODE", "Descriptive Name"="TV Trigger Mode", "Data Type"=0, "Command"="TRIGger1:TV:MODE", "Access"=2, "Range Table"="rsscope_rngTVTriggerMode", "Read Callback"="", "Write Callback"="", "Supported Models"="", "Instrument Options"="", "Flags"=0, "Help"="Selects the lines or fields on which the instrument can trigger. Available modes depend on the scanning system.\n\nAvailable Repeated Capabilities:\nNone\n\nRemote-control command(s):\nTRIGger<m>:TV:MODE"}, {"Level"=3, "Class Only"=FALSE, "Identifier"="RSSCOPE_ATTR_TV_TRIGGER_LINE_NUMBER", "Descriptive Name"="TV Trigger Line Number", "Data Type"=0, "Command"="TRIG:TV:LINE", "Access"=2, "Range Table"="rsscope_rngLineNumber", "Read Callback"="", "Write Callback"="", "Supported Models"="", "Instrument Options"="", "Flags"=0, "Help"="Sets an exact line number if Trigger Event is set to LINE.\n\nAvailable Repeated Capabilities:\nNone\n\nRemote-control command(s):\nTRIGger<m>:TV:LINE"}, {"Level"=3, "Class Only"=FALSE, "Identifier"="RSSCOPE_ATTR_TV_TRIGGER_FIELD", "Descriptive Name"="TV Trigger Field", "Data Type"=0, "Command"="TRIG:TV:LFI", "Access"=2, "Range Table"="rsscope_rngTVTriggerField", "Read Callback"="", "Write Callback"="", "Supported Models"="", "Instrument Options"="", "Flags"=0, "Help"="Sets the field in which the line number is counted. This control is only relevant for NTSC signals\n\nAvailable Repeated Capabilities:\nNone\n\nRemote-control command(s):\nTRIGger<m>:TV:LFIeld"}, {"Level"=3, "Class Only"=FALSE, "Identifier"="RSSCOPE_ATTR_TV_TRIGGER_POLARITY", "Descriptive Name"="TV Trigger Polarity", "Data Type"=0, "Command"="TRIG:TV:POL", "Access"=2, "Range Table"="rsscope_rngPolarity", "Read Callback"="", "Write Callback"="", "Supported Models"="", "Instrument Options"="", "Flags"=0, "Help"="Sets the polarity of the signal. Note that the sync pulse has the opposite polarity, for example, a positive signal has a negative sync pulse.\n\nAvailable Repeated Capabilities:\nNone\n\nRemote-control command(s):\nTRIGger<m>:TV:POLarity"}, {"Level"=3, "Class Only"=FALSE, "Identifier"="RSSCOPE_ATTR_TV_TRIGGER_PULSE_TYPE", "Descriptive Name"="TV Trigger Pulse Type", "Data Type"=0, "Command"="TRIGger1:TV:CUST:STYP", "Access"=2, "Range Table"="rsscope_rngTVTriggerPulseType", "Read Callback"="", "Write Callback"="", "Supported Models"="", "Instrument Options"="", "Flags"=0, "Help"="Sets the type of the sync pulse.\n\nAvailable Repeated Capabilities:\nNone\n\nRemote-control command(s):\nTRIGger<m>:TV:CUSTom:STYPe"}, {"Level"=3, "Class Only"=FALSE, "Identifier"="RSSCOPE_ATTR_TV_TRIGGER_LINE_PERIOD", "Descriptive Name"="TV Trigger Line Period", "Data Type"=1, "Command"="TRIGger1:TV:CUST:LDUR", "Access"=2, "Range Table"="rsscope_rngTVLinePeriod", "Read Callback"="", "Write Callback"="", "Supported Models"="", 
